vi "Read Discrete Inputs1.vi"(7 "Unit_ID":T1={"Protocol ID"=0, "Unit ID"=1}, 8 "error in (no error)":errorcluster, 9 "number of discrete inputs":u16, 10 "starting address":u16, 11 "Modbus master in":refnum<class "TCP.lvclass">) -> (0 "error out":errorcluster, 2 "discrete input values":bool[](array[boolean]), 3 "Modbus master out":refnum<class "TCP.lvclass">)   [LabVIEW 2019, in "NI_modbus_upd.lvlib"]
doc: "Reads values from contiguous discrete inputs. The maximum number of discrete inputs this VI can read is 2,000."
uses:
  NI_modbus_upd.lvlib
  TCP/TCP.lvclass
  Ctl/Unit_ID.ctl
  TCP/TCP.lvclass/TCP.ctl
  Utility/Bytes to Bits1.vi
  Function code mismatch error1.vi
  Error Generator1.vi
  Read ADU Packet Master.vi
  Write ADU Packet Master.vi
  Modbus Data Unit (PDU)/Construct PDU1.vi
  Modbus Data Unit (PDU)/Unflatten to PDU1.vi
  TCP/Protocol Read.vi
  TCP/Protocol Write.vi
  <vilib>/Utility/error.llb/Clear Errors.vi
  Modbus Data Unit (PDU)/Deconstruct PDU1.vi
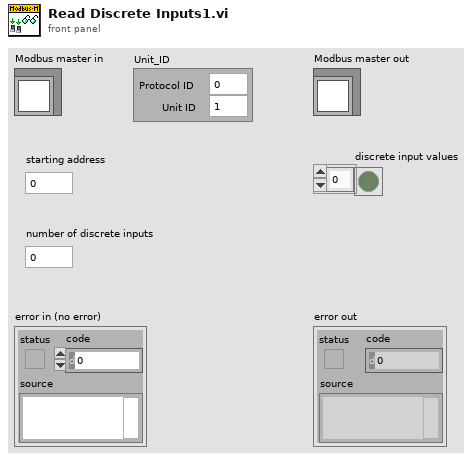
[diagram p1: front panel]
types:
  T1 = typedef "NI_modbus_upd.lvlib/Unit_ID.ctl" = cluster{"Protocol ID":u16, "Unit ID":u8}
  T2 = typedef "NI_modbus_upd.lvlib/MB Modbus Data Unit.ctl" = cluster{"function":T3, "Data":u8[]}
  T3 = typedef "NI_modbus_upd.lvlib/Function.ctl" = u8
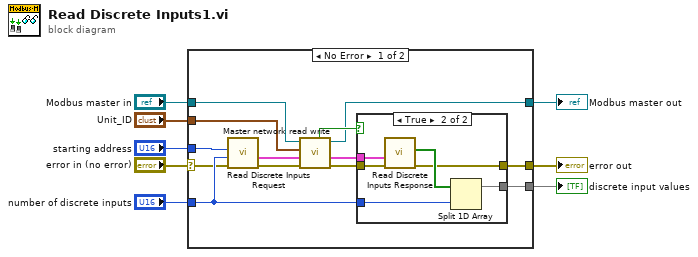
[diagram p0: block diagram]
diagram:
  n1 = case shown="No Error" "error in (no error)" {
    selector: "error in (no error)" -> [w16 w30]
    tunnel: [w17 w30] -> w2
    tunnel: [w12 w29] -> w4
    tunnel: "Modbus master in" -> [w15 w29]
    tunnel: "starting address" -> [w21 _]
    tunnel: "number of discrete inputs" -> [w20 _]
    tunnel: [w19 _] -> w3
    tunnel: "Unit_ID" -> [w10 _]
    frame No Error {
      n2 = call "Read Discrete Inputs Request.vi"("error in (no error)"=w16, "number of inputs"=w20, "starting address"=w21) -> ("error out"=w14:errorcluster, "Modbus Data Unit out"=w9:T2)  [unwired: 7 in]
      n3 = call "Master network read write.vi"("error in (no error)"=w14, "Modbus Data Unit"=w9, "Unit_ID"=w10, "TCP in"=w15) -> ("error out"=w18:errorcluster, "Modbus data unit out"=w11:T2, "TCP out"=w12:refnum<class "TCP.lvclass">, "PDU valid?"=w13:bool)  [unwired: 4 in]
      n4 = case shown="True" w13 {
        tunnel: w20 -> [_ w28]
        tunnel: [_ w27] -> w19
        tunnel: w18 -> [w22 w25]
        tunnel: [w22 w24] -> w17
        tunnel: w11 -> [_ w23]
        frame False {
        }
        frame True {
          n5 = call "Read Discrete Inputs Response.vi"("error in (no error)"=w25, "Modbus Data Unit in"=w23) -> ("error out"=w24:errorcluster, "data"=w26:bool[])  [unwired: 8 in]
          n6 = Split 1D Array(array=w26, index=w28) -> (first subarray=w27:bool[])  [unwired: 1 out]
        }
      }
    }
    frame Error {
    }
  }
  "error out" <- w2
  "Modbus master out" <- w4
  "discrete input values" <- w3
